vi "MGI Get Cluster Value.vi"(8 "Error In":errorcluster, 9 "Flat? (F)":bool, 10 "Name":string, 11 "Cluster In":variant) -> (0 "Error Out":errorcluster, 1 "Found?":bool, 3 "Value":variant)   [LabVIEW 2016]
doc: "This VI is designed to return the value of an element in a cluster (as a variant) based on the name provided. If there are multiple fields with the same name, only the first will be returned. Setting <B>Flat?</B> to True avoids searching in subclusters.\n\nAuthored by Robert C. Mortensen\nsupport@mooregoodideas.com\nwww.mooregoodideas.com\n\nCopyright (c) 2010, Moore Good Ideas, Inc.\n\nAll rights reserved.\n\nRedistribution and use in source and binary forms, with or without modification, are permitted provided that the following conditions are met:\n\n * Redistributions of source code must retain the above copyright notice, this list of conditions and the following disclaimer.\n * Redistributions in binary form must reproduce the above copyright notice, this list of conditions and the following disclaimer in the documentation and/or other materials provided with the distribution.\n * Neither the name of Moore Good Ideas, Inc. nor the names of its contributors may be used to endorse or promote products derived from this software without specific prior written permission.\n\nTHIS SOFTWARE IS PROVIDED BY THE COPYRIGHT HOLDERS AND CONTRIBUTORS \"AS IS\" AND ANY EXPRESS OR IMPLIED WARRANTIES, INCLUDING, BUT NOT LIMITED TO, THE IMPLIED WARRANTIES OF MERCHANTABILITY AND FITNESS FOR A PARTICULAR PURPOSE ARE DISCLAIMED. IN NO EVENT SHALL THE COPYRIGHT OWNER OR CONTRIBUTORS BE LIABLE FOR ANY DIRECT, INDIRECT, INCIDENTAL, SPECIAL, EXEMPLARY, OR CONSEQUENTIAL DAMAGES (INCLUDING, BUT NOT LIMITED TO, PROCUREMENT OF SUBSTITUTE GOODS OR SERVICES; LOSS OF USE, DATA, OR PROFITS; OR BUSINESS INTERRUPTION) HOWEVER CAUSED AND ON ANY THEORY OF LIABILITY, WHETHER IN CONTRACT, STRICT LIABILITY, OR TORT (INCLUDING NEGLIGENCE OR OTHERWISE) ARISING IN ANY WAY OUT OF THE USE OF THIS SOFTWARE, EVEN IF ADVISED OF THE POSSIBILITY OF SUCH DAMAGE."
uses:
  <vilib>/Utility/VariantDataType/VariantType.lvlib
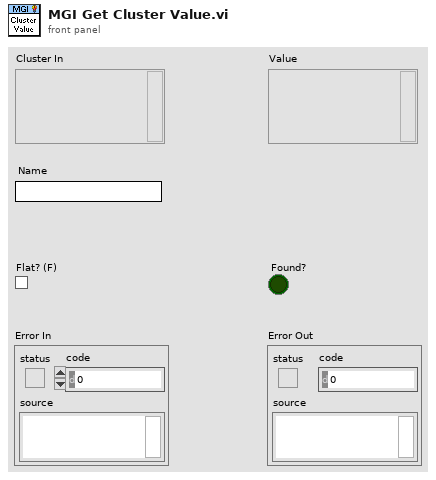
[diagram p1: front panel]
types:
  T1 = typedef "VariantType.lvlib/Type.ctl" = enum8{"Invalid Type", "Void", "I8", "I16", "I32", "I64", "U8", "U16", "U32", "U64", "Single Float", "Double Float", "Extended Float", "Single Complex", "Double Complex", "Extended Complex", "Enum U8", "Enum U16", "Enum U32", "Enum U64", "Single Float With Unit", "Double Float With Unit", "Extended Float With Unit", "Single Complex with Unit", "Double Complex with Unit", "Extended Complex with Unit", "Boolean", "String", "Path", "Picture", "Tag", "Array", "Cluster", "Variant", "LV Variant", "Waveform", "Timestamp", "Digital Waveform", "Digital Data", "ExpressData", "Refnum", "External Data", "VI", "Poly VI", "LabVIEW Class Instance", "Fixed Point"}
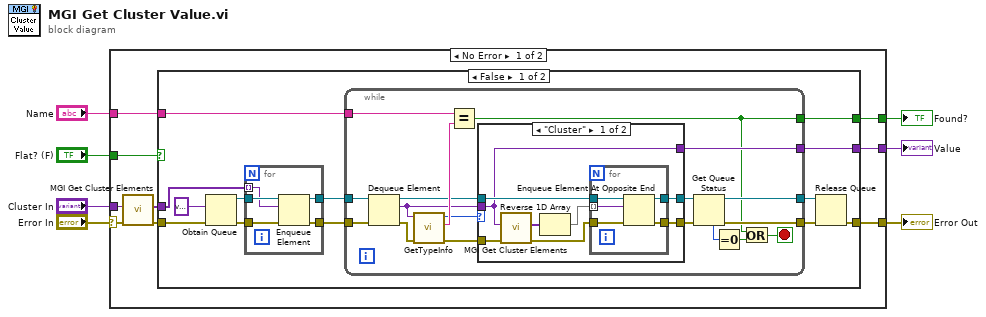
[diagram p0: block diagram]
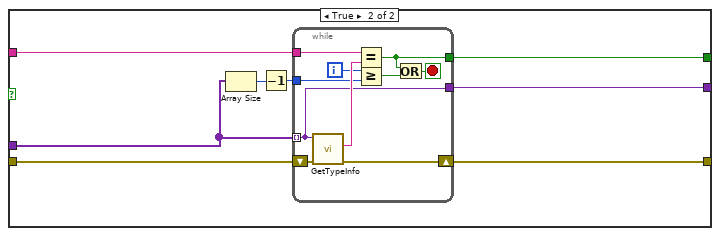
[diagram p3: hidden frame]
diagram:
  n1 = case shown="No Error" "Error In" {
    selector: "Error In" -> [w8 w87]
    tunnel: "Cluster In" -> [w16 _]
    tunnel: "Name" -> [w13 _]
    tunnel: [w12 w87] -> w5
    tunnel: [w11 _] -> w4
    tunnel: [w10 _] -> w3
    tunnel: "Flat? (F)" -> [w9 _]
    frame No Error {
      n2 = call <userlib>:"MGI Get Cluster Elements.vi"("Error In"=w8, "Cluster"=w16) -> ("Error Out"=w15:errorcluster, "Cluster Elements"=w14:variant[])  [unwired: 8 in]
      n3 = case shown="False" w9 {
        tunnel: w15 -> [w29 w76]
        tunnel: w14 -> [w26 w70]
        tunnel: w13 -> [w22 w74]
        tunnel: [w19 w72] -> w12
        tunnel: [w18 w73] -> w11
        tunnel: [w17 w75] -> w10
        frame False {
          n4 = Obtain Queue(element data type=variant, error in (no error)=w29) -> (queue out=w27:refnum<queue>, error out=w28:errorcluster)  [unwired: 3 in, 1 out]
          n5 = for {
            tunnel: w28 -> [w68]
            tunnel: w27 -> [w67]
            tunnel: w26 -> [w66] mode=indexing
            tunnel: [w65] -> w23
            tunnel: [w64] -> w24
            n6 = Enqueue Element(queue=w67, element=w66, error in (no error)=w68) -> (queue out=w64:refnum<queue>, error out=w65:errorcluster)  [unwired: 1 in, 1 out]
          }
          n7 = while {
            tunnel: w24 -> [w46]
            tunnel: w23 -> [w47]
            tunnel: w22 -> [w40]
            tunnel: [w33] -> w21
            tunnel: [w32] -> w20
            tunnel: [w31] -> w17
            tunnel: [w30] -> w18
            stop <- w43 stop-if-true
            n8 = Dequeue Element(queue=w46, error in (no error)=w47) -> (queue out=w38:refnum<queue>, element=w34:variant, error out=w42:errorcluster)  [unwired: 1 in, 1 out]
            n9 = call <vilib>:"GetTypeInfo.vi"("error in (no error)"=w42, "Variant"=w34) -> ("error out"=w37:errorcluster, "Name"=w41:string, "Type Enum"=w39:T1)  [unwired: 5 in, 2 out]
            n10 = Equal?(x=w40, y=w41) -> (x = y?=w30:bool)
            n11 = case shown="\"Cluster\"" w39 {
              tunnel: w38 -> [w50 w63]
              tunnel: w37 -> [w55 w62]
              tunnel: w34 -> [w48 w61]
              tunnel: [w53 w62] -> w36
              tunnel: [w52 w63] -> w35
              tunnel: [w48 w61] -> w31
              frame "Cluster" {
                n12 = call <userlib>:"MGI Get Cluster Elements.vi"("Error In"=w55, "Cluster"=w48) -> ("Error Out"=w51:errorcluster, "Cluster Elements"=w54:variant[])  [unwired: 8 in]
                n13 = Reverse 1D Array(array=w54) -> (reversed array=w49:variant[])
                n14 = for {
                  tunnel: w51 -> [w60]
                  tunnel: w50 -> [w59]
                  tunnel: w49 -> [w58] mode=indexing
                  tunnel: [w57] -> w53
                  tunnel: [w56] -> w52
                  n15 = Enqueue Element At Opposite End(queue=w59, element=w58, error in (no error)=w60) -> (queue out=w56:refnum<queue>, error out=w57:errorcluster)  [unwired: 1 in, 1 out]
                }
              }
              frame Default {
              }
            }
            n16 = Get Queue Status(queue=w35, error in (no error)=w36) -> (queue out=w32:refnum<queue>, error out=w33:errorcluster, # elements in queue=w45:i32)  [unwired: 1 in, 5 out]
            n17 = Equal To 0?(x=w45) -> (x = 0?=w44:bool)
            n18 = Or(x=w30, y=w44) -> (x .or. y?=w43:bool)
          }
          n19 = Release Queue(queue=w20, error in (no error)=w21) -> (error out=w19:errorcluster)  [unwired: 1 in, 2 out]
        }
        frame True {
          n20 = Array Size(array=w70) -> (size(s)=w71:i32)
          n21 = Decrement(x=w71) -> (x-1=w69:i32)
          n22 = while {
            tunnel: w70 -> [w84] mode=indexing
            tunnel: [w84] -> w75
            tunnel: w74 -> [w83]
            tunnel: [w80] -> w73
            shift-right: [w82] -> w72
            shift-left: w76 -> [w86]
            tunnel: w69 -> [w78]
            i -> [w77]
            stop <- w81 stop-if-true
            n23 = call <vilib>:"GetTypeInfo.vi"("error in (no error)"=w86, "Variant"=w84) -> ("error out"=w82:errorcluster, "Name"=w85:string)  [unwired: 5 in, 3 out]
            n24 = Equal?(x=w83, y=w85) -> (x = y?=w80:bool)
            n25 = Greater Or Equal?(x=w77, y=w78) -> (x >= y?=w79:bool)
            n26 = Or(x=w80, y=w79) -> (x .or. y?=w81:bool)
          }
        }
      }
    }
    frame Error {
    }
  }
  "Error Out" <- w5
  "Value" <- w3
  "Found?" <- w4
